vi "Draw Flat Bottom Filled Triangle.vi"(4 "Fill Colour":u32(colorbox), 6 "Enable Alpha Blending (F)":bool, 7 "Alpha":dbl, 8 "Vertex 3":T1={"Position"={"x"=0.0, "y"=0.0, "z"=0.0}, "UV"={"u"=0.0, "v"=0.0}, "Colour"=12517256} {"UV"."v" min=0 max=1 step=0.1; "UV"."u" min=0 max=1 step=0.1}, 9 "Vertex 2":T1={"Position"={"x"=0.0, "y"=0.0, "z"=0.0}, "UV"={"u"=0.0, "v"=0.0}, "Colour"=12517256} {"UV"."v" min=0 max=1 step=0.1; "UV"."u" min=0 max=1 step=0.1}, 10 "Vertex 1":T1={"Position"={"x"=0.0, "y"=0.0, "z"=0.0}, "UV"={"u"=0.0, "v"=0.0}, "Colour"=12517256} {"UV"."v" min=0 max=1 step=0.1; "UV"."u" min=0 max=1 step=0.1}, 11 "Pixel Data in":u32[][](array[numeric])) -> (3 "Pixel Data out":u32[][](array[numeric]))   [LabVIEW 2020, in "Raster (FPGA).lvlib"]
uses:
  Raster (FPGA).lvlib
  3D/Vertex.ctl
  3D/Vector 3D.ctl
  UV.ctl
  Point 2D (I32).ctl
  Method.ctl
  c0c82237-b583-4fc1-b44f-40d02a28ecfd.vi
  53435b12-820c-4aea-aec4-7de16a894549.vi
  <vilib>/Utility/High Resolution Relative Seconds.vi
  Global 1.vi
  <vilib>/Utility/colorconv.llb/Color to RGB.vi
  <vilib>/Utility/colorconv.llb/RGB to Color.vi
  3D/3D (FPGA).lvlib
panel:
  out "Delta Time [s]":dbl format="%.3p"
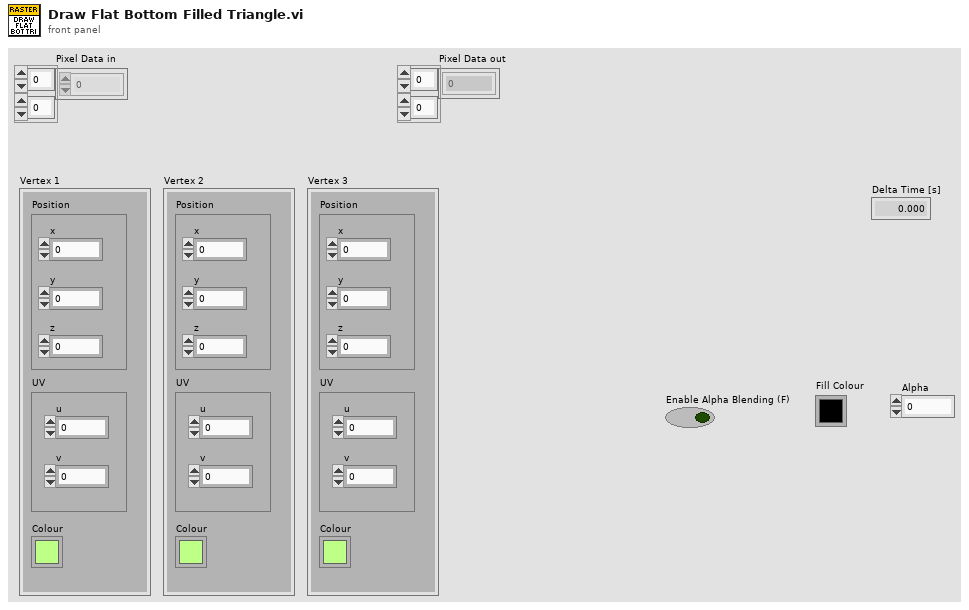
[diagram p1: front panel]
types:
  T1 = typedef "3D (FPGA).lvlib/Vertex.ctl" = cluster{"Position":T2, "UV":T3, "Colour":u32}
  T2 = typedef "3D (FPGA).lvlib/Vector 3D.ctl" = cluster{"x":sgl, "y":sgl, "z":sgl}
  T3 = typedef "Raster (FPGA).lvlib/UV.ctl" = cluster{"u":sgl, "v":sgl}
  T4 = typedef "Raster (FPGA).lvlib/Point 2D (I32).ctl" = cluster{"x":i32, "y":i32}
  T5 = typedef "Raster (FPGA).lvlib/Method.ctl" = enum16{"Per item", "Row", "Replace Array Subset", "MoveBlock", " MoveBlock2 "}
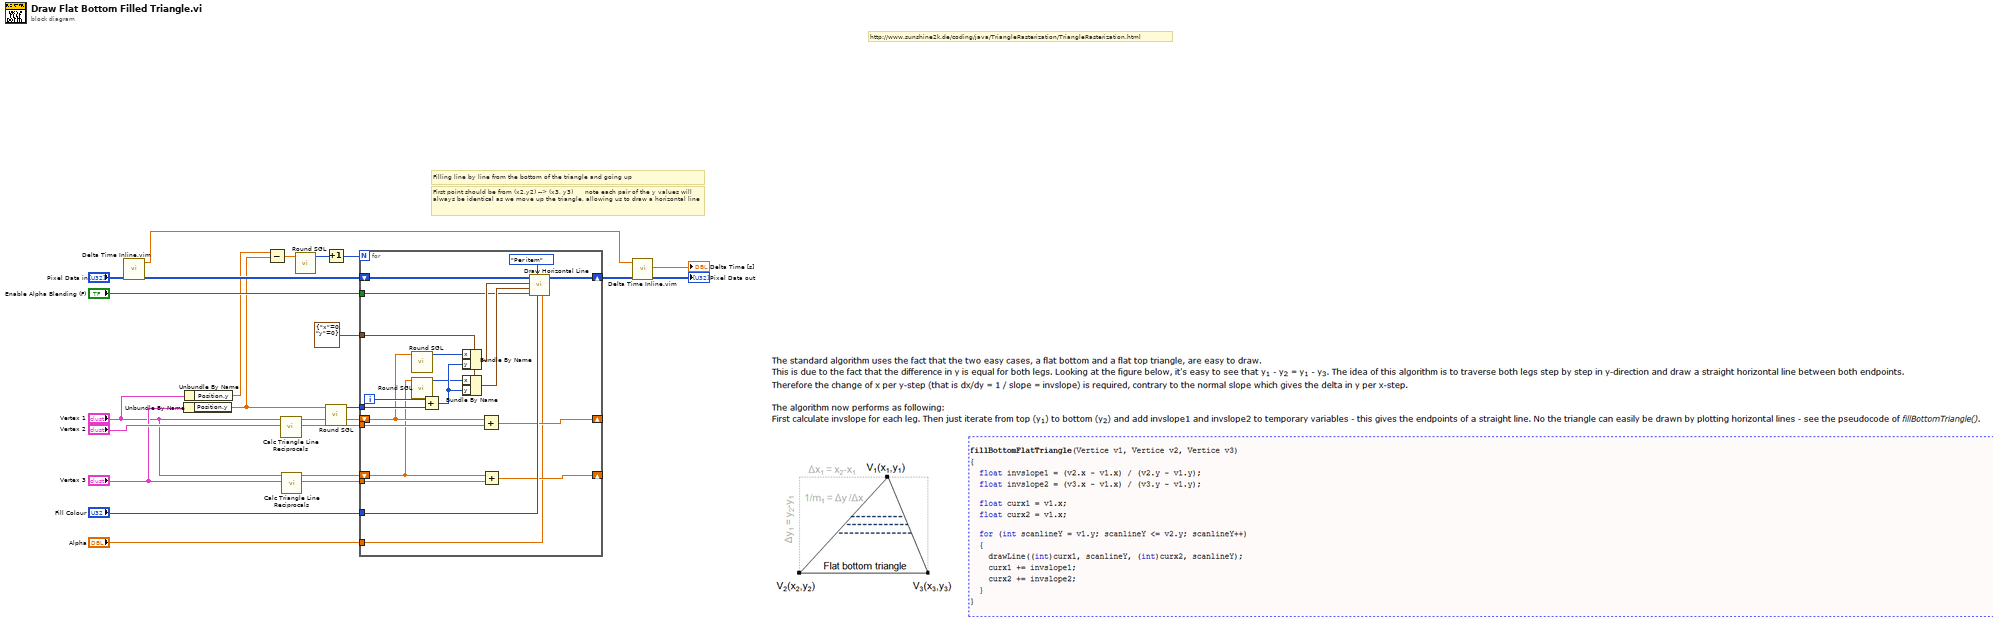
[diagram p0: block diagram]
diagram:
  # "First point should be from (x2,y2) --> (x3, y3)      note each pair of the y values will always be identical as we move up the triangle, allowing us to draw a horizontal line"
  # "Filling line by line from the bottom of the triangle and going up"
  # "http://www.sunshine2k.de/coding/java/TriangleRasterization/TriangleRasterization.html"
  n1 = call "Delta Time Inline.vim"("value in"="Pixel Data in") -> ("value out"=w16:u32[][], "Relative Seconds out [s]"=w13:dbl)  [unwired: 8 in, 1 out]
  n2 = Unbundle By Name("Vertex 3") -> ("Position.y"=w2:sgl)
  n3 = Unbundle By Name("Vertex 1") -> ("Position.y"=w3:sgl)
  n4 = Subtract(x=w3, y=w2) -> (x-y=w10:sgl)
  n5 = call "Calc Triangle Line Reciprocals.vi"("Vertex 2"="Vertex 2", "Vertex 1"="Vertex 1") -> ("Delta x"=w21:sgl, "Starting x"=w20:sgl)  [unwired: 8 in]
  n6 = call "Calc Triangle Line Reciprocals.vi"("Vertex 2"="Vertex 3", "Vertex 1"="Vertex 1") -> ("Delta x"=w6:sgl, "Starting x"=w7:sgl)  [unwired: 8 in]
  n7 = call "Round SGL.vi"("SGL"=w10) -> ("I32"=w9:i32)  [unwired: 10 in]
  n8 = Increment(x=w9) -> (x+1=w11:i32)
  n9 = call "Round SGL.vi"("SGL"=w2) -> ("I32"=w8:i32)  [unwired: 10 in]
  n10 = for {
    N: w11 -> [_]
    tunnel: T4 {"x"=0, "y"=0} ("Point 1") -> [w43]
    tunnel: "Fill Colour" -> [w40]
    shift-right: [w34] -> _
    shift-left: w20 -> [w27]
    shift-right: [w35] -> _
    shift-left: w7 -> [w25]
    tunnel: w8 -> [w37]
    tunnel: w21 -> [w36]
    tunnel: w6 -> [w33]
    shift-right: [w31] -> w15
    shift-left: w16 -> [w32]
    tunnel: "Enable Alpha Blending (F)" -> [w29]
    tunnel: "Alpha" -> [w28]
    i -> [w39]
    n11 = call "Round SGL.vi"("SGL"=w27) -> ("I32"=w26:i32)  [unwired: 10 in]
    n12 = call "Round SGL.vi"("SGL"=w25) -> ("I32"=w24:i32)  [unwired: 10 in]
    n13 = Add(x=w39, y=w37) -> (x+y=w38:i32)
    n14 = Bundle By Name(cluster=w43, "x"=w26, "y"=w38) -> (w42:T4)
    n15 = Bundle By Name(cluster=w43, "x"=w24, "y"=w38) -> (w41:T4)
    n16 = Add(x=w27, y=w36) -> (x+y=w34:sgl)
    n17 = Add(x=w25, y=w33) -> (x+y=w35:sgl)
    n18 = call "Draw Horizontal Line.vi"("Alpha"=w28, "Colour"=w40, "Method"=Method."Per item", "Enable Alpha Blending (F)"=w29, "Point 2"=w41, "Point 1"=w42, "Pixel Data in"=w32) -> ("Pixel Data out"=w31:u32[][])  [unwired: 4 in]
  }
  n19 = call "Delta Time Inline.vim"("value in"=w15, "Relative Seconds in [s]"=w13) -> ("value out"=→"Pixel Data out":u32[][], "Delta Time [s]"=→"Delta Time [s]":dbl)  [unwired: 7 in, 1 out]
